vi "Set Blower Level.vi"(8 "error in":errorcluster, 10 "Level":u8, 11 "Neph in":refnum<class "Nephelometer.lvclass">) -> (0 "error out":errorcluster, 3 "Neph out":refnum<class "Nephelometer.lvclass">)   [LabVIEW 2014, in "Nephelometer.lvclass"]
uses:
  Nephelometer.lvclass
  Reusable/Session APIs/Serial/Serial Session.lvclass
  Nephelometer.lvclass/Nephelometer.ctl
  Accessors/Read Session Handle.vi
  <userlib>/_Session Fwk/Session - Root.lvclass
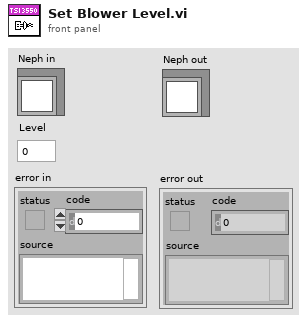
[diagram p1: front panel]
types:
  T1 = typedef "Session - Root.lvclass/Session Handle.ctl" = refnum<data-value>
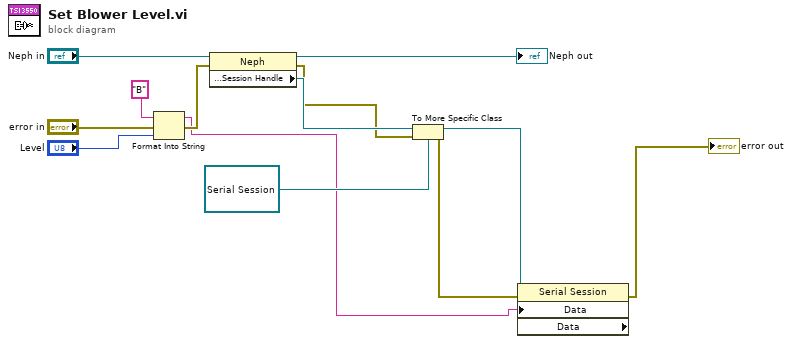
[diagram p0: block diagram]
diagram:
  n1 = Format Into String(initial string="B", error in="error in", "Level") -> (resulting string=w2:string, error out=w9:errorcluster)  [unwired: 1 in]
  n2 = property class="Neph"(reference="Neph in", error in=w9) -> (reference out=→"Neph out":refnum<class "Nephelometer.lvclass">, error out=w3:errorcluster, "Accessors:Session Handle"=w4:T1)
  n3 = To More Specific Class(target class=refnum<data-value> refnum ("Session Handle"), reference=w4, error in=w3) -> (specific class reference=w6:refnum<data-value>, error out=w5:errorcluster)
  n4 = property class="Serial Session" props=["Data", "Data"](reference=w6, error in=w5, "Data"=w2) -> (error out=→"error out":errorcluster)  [unwired: 2 out]
